vi "Dial_Gauge.vi"() -> ()   [LabVIEW 2024]
uses:
  <vilib>/Utility/miscctls.llb/LVRowAndColumnTypeDef.ctl
panel:
  out "nominal":dbl format="%.1f"
  out "Edit Position":T1
  in  "Table Control":string[][](table)
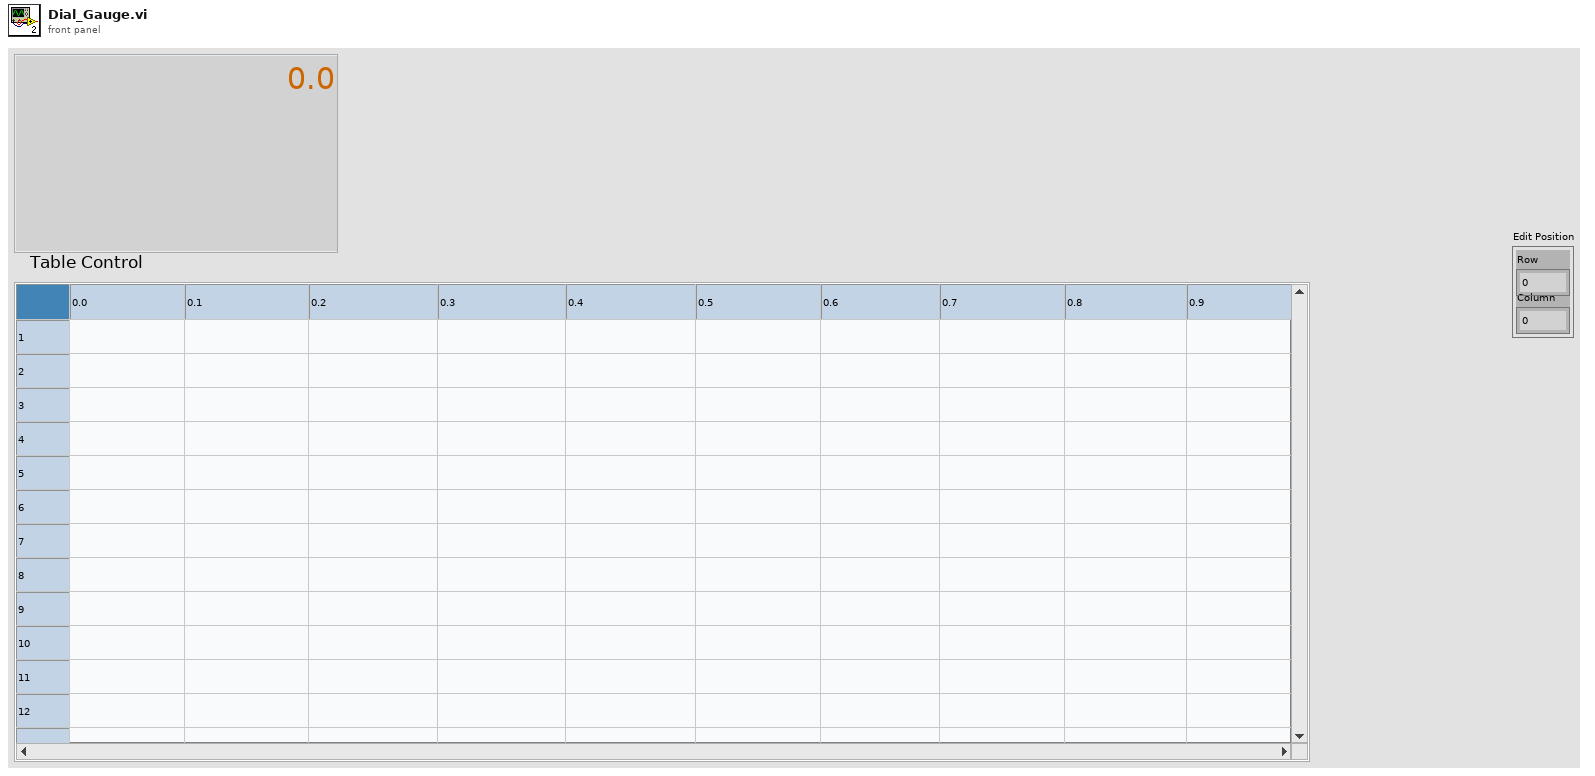
[diagram p1: front panel]
types:
  T1 = typedef "LVRowAndColumnTypeDef.ctl" = cluster{"Row":i32, "Column":i32}
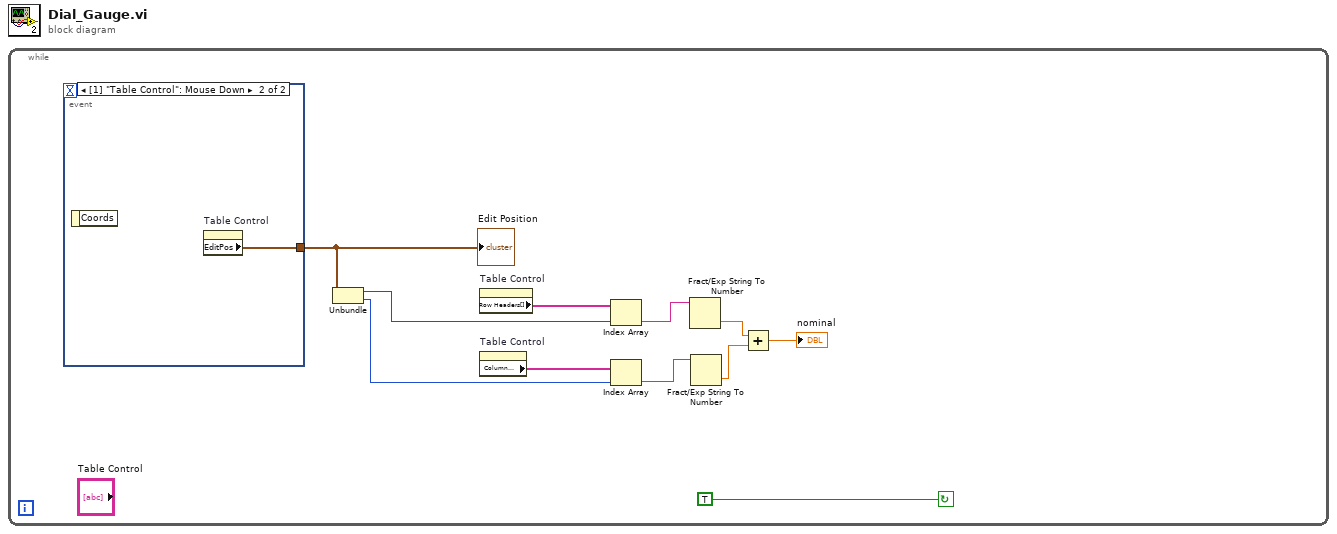
[diagram p0: block diagram]
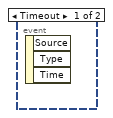
[diagram p2: hidden frame]
diagram:
  n1 = while {
    stop <- TRUE continue-if-true
    n2 = event shown="[1] \"Table Control\": Mouse Down" {
      selector: _ -> [_ _]
      dyn-events: _ -> [_ _]
      timeout: _ -> [_ _]
      tunnel: [_ w12] -> w1
      event Timeout {
        n3 = event-data() -> ()  [unwired: 1 in, 3 out]
      }
      event "Table Control": Mouse Down {
        n4 = event-data() -> ()  [unwired: 1 in, 1 out]
        n5 = property on="Table Control" class="Tbl (strict)"() -> ("EditPos"=w12:T1)  [unwired: 2 in, 2 out]
      }
    }
    "Edit Position" <- w1
    n6 = Unbundle(w1) -> ("Row"=w3:i32, "Column"=w5:i32)
    n7 = property on="Table Control" class="Tbl (strict)"() -> ("Row Headers[]"=w2:string[])  [unwired: 2 in, 2 out]
    n8 = property on="Table Control" class="Tbl (strict)"() -> ("Column Headers[]"=w4:string[])  [unwired: 2 in, 2 out]
    n9 = Index Array(array=w2, index=w3) -> (element=w6:string)
    n10 = Index Array(array=w4, index=w5) -> (element=w7:string)
    n11 = Fract/Exp String To Number(string=w6) -> (number=w8:dbl)  [unwired: 3 in, 1 out]
    n12 = Fract/Exp String To Number(string=w7) -> (number=w9:dbl)  [unwired: 3 in, 1 out]
    n13 = Add(x=w8, y=w9) -> (x+y=→"nominal":dbl)
  }
